vi "Test Flatten.vi"() -> ()   [LabVIEW 2021]
uses:
  ChannelCommon/typedef/FIFO Header.ctl
  ChannelCommon/typedef/Datatype Waveform.ctl
  ChannelCommon/typedef/TimeStamps.ctl
  CIF_NIChn_FIFO_DAQ.lvclass
  D:/dev/Packages/Channel_Manager/src/CIF_NIChn/FIFO_U8/CIF_NIChn_Fifo_U8.lvclass
  D:/dev/Packages/Channel_Manager/src/CIFChannels/CIFChannels.lvclass
  CIFChannels/Typedef/Direction.ctl
  FIFO_U8/CIF_NIChn_Fifo_U8.lvclass/CIF_NIChn_Fifo_U8.ctl
  CIFChannels/CIFChannels.lvclass/CIFChannels.ctl
  <vilib>/CIF Foundation/CIF Utilities/Statistics/I64/Stats_I64_CIF_U.lvclass/Stats_I64_CIF_U.ctl
  CIFChannels/Utilities/Update Flatten Benchmark.vi
  SubVIs/Flatten.vi/587a020d-d764-4ff7-9451-6b801beca2fa.vi
  SubVIs/Flatten.vi/b511efe2-f594-4971-95dc-73ac55586360.vi
  ChannelCommon/CIFFIFO/Flatten/Waveform Flatten.vi
  FIFO_U8/Accessors/Read Payload.vi
  FIFO_U8/Accessors/Write Payload.vi
  SubVIs/Unflatten.vi/4ab41953-a001-49d2-beab-55370b6c3c42.vi
  SubVIs/Unflatten.vi/7cd889b7-face-4678-a9e3-2692853b6930.vi
  ChannelCommon/CIFFIFO/Flatten/Waveform Unflatten.vi
  CIFChannels/Accessors/Write FIFO Timeout.vi
  <vilib>/CIF Foundation/CIF Utilities/Statistics/I64/X1 minus X0.vi
  <vilib>/CIF Foundation/CIF Utilities/Time/System Time/Get System Time.vi
  <vilib>/CIF Foundation/CIF Utilities/DataTypes/Flatten I64.vi
  ChannelCommon/CIFFIFO/Flatten/Waveform Flatten.vi/be24e584-1bb9-4ddb-b1ad-5fa4498d0a1e.vi
  <vilib>/CIF Foundation/CIF Utilities/DataTypes/Flatten U64.vi
  CIFChannels/Utilities/Create Flattened FIFO Header.vi
  ChannelCommon/Utilities/Unflatten Header.vi
  <vilib>/CIF Foundation/CIF Utilities/DataTypes/Unflatten I64.vi
  <vilib>/CIF Foundation/CIF Utilities/Statistics/I64/X1 minus X0.vi/dfabcf33-0dbc-4041-80a5-3dc0c86d2989.vi
  <vilib>/CIF Foundation/CIF Utilities/Time/System Time/LabVIEW Time to TAI Time.vi
  ChannelCommon/CIFFIFO/Flatten/Waveform Flatten.vi/be24e584-1bb9-4ddb-b1ad-5fa4498d0a1e.vi/c28b0ead-42ad-4072-80a2-aca7f2bd7ce3.vi
  ChannelCommon/Utilities/Flatten Header.vi
  CIFChannels/Utilities/Update FIFO Header.vi
  <vilib>/CIF Foundation/CIF Utilities/DataTypes/Unflatten U64.vi
  ChannelCommon/Utilities/Add Error.vi
  <vilib>/CIF Foundation/CIF Utilities/Statistics/I64/X1 minus X0.vi/dfabcf33-0dbc-4041-80a5-3dc0c86d2989.vi/9eb60a9a-770f-4d2d-8b3f-8465c267ecc9.vi
  <vilib>/CIF Foundation/CIF Utilities/Errors/Append Error Location.vi
  CIFChannels/CIFChannels.lvclass
  ChannelCommon/ChannelCommon.lvlib
panel:
  out "Pass":bool
  out "error out":errorcluster
  in  "FIFO Timestamps":T1={"ClockID"=2, "T0"=432, "T_Out"=543}
  out "Data out":T2[](array[typedef])=[{"measurement"=[0.0, 0.0, 0.0, 0.0, 0.0, 0.0, 0.0, 3.14], "dT"=0.01, "Timestamp"=498, "Read Lock"=FALSE}, {"measurement"=[0.0, 0.0, 0.0, 0.0, 0.0, 0.0, 0.0, 9.8], "dT"=0.12, "Timestamp"=12345, "Read Lock"=FALSE}]
  in  "Data In":T2[](array[typedef])=[{"measurement"=[0.0, 0.0, 0.0, 0.0, 0.0, 0.0, 0.0, 3.14], "dT"=0.01, "Timestamp"=498, "Read Lock"=FALSE}, {"measurement"=[0.0, 0.0, 0.0, 0.0, 0.0, 0.0, 0.0, 9.8], "dT"=0.12, "Timestamp"=12345, "Read Lock"=FALSE}]
  out "Header":T3={"Length"=57, "T0"=432, "T_Out"=543, "T_Tx"=1727639110950812000, "Ctr"=1, "ClockID"=2}
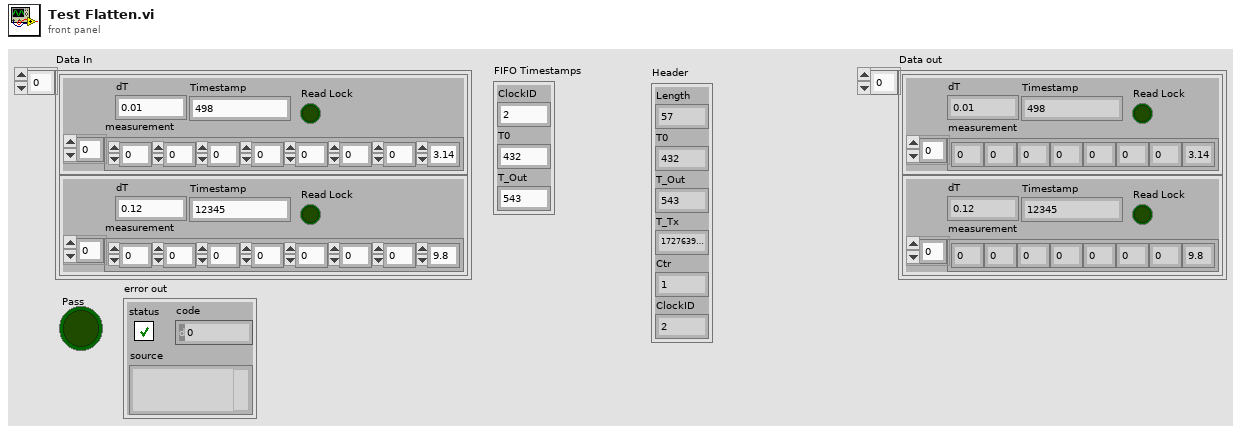
[diagram p1: front panel]
types:
  T1 = typedef "ChannelCommon.lvlib/TimeStamps.ctl" = cluster{"ClockID":u8, "T0":i64, "T_Out":i64}
  T2 = typedef "ChannelCommon.lvlib/Datatype Waveform.ctl" = cluster{"measurement":dbl[], "dT":dbl, "Timestamp":i64, "Read Lock":bool}
  T3 = typedef "ChannelCommon.lvlib/FIFO Header.ctl" = cluster{"Length":u64, "T0":i64, "T_Out":i64, "T_Tx":i64, "Ctr":u64, "ClockID":u8}
  T4 = typedef "CIFChannels.lvclass/Direction.ctl" = enum16{"Publisher", "Subscriber"}
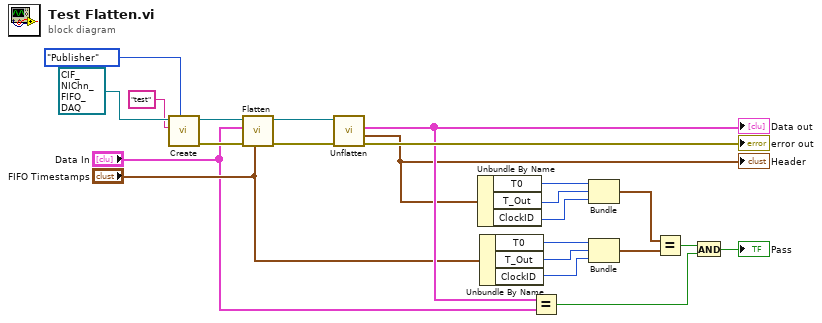
[diagram p0: block diagram]
diagram:
  n1 = call-dynamic "Create.vi"("Direction"=Direction."Publisher", "Name"="test", "CIFFIFO in"=refnum<class "CIF_NIChn_FIFO_DAQ.lvclass"> refnum ("CIF_NIChn_Fifo_Power.lvclass")) -> ("error out"=w17:errorcluster, "CIFFIFO out"=w19:refnum<class "CIF_NIChn_FIFO_DAQ.lvclass">)  [unwired: 7 in]
  n2 = call "Flatten.vi"("FIFO Timestamps"="FIFO Timestamps", "error in (no error)"=w17, "Data In"="Data In", "CIF_NIChn_FIFO_DAQ in"=w19) -> ("error out"=w18:errorcluster, "CIF_NIChn_FIFO_DAQ out"=w23:refnum<class "CIF_NIChn_FIFO_DAQ.lvclass">)  [unwired: 5 in, 1 out]
  n3 = call "Unflatten.vi"("error in (no error)"=w18, "CIF_NIChn_FIFO_DAQ in"=w23) -> ("error out"=→"error out":errorcluster, "Header"=w14:T3, "DAQ Out"=w15:T2[])  [unwired: 6 in, 1 out]
  "Header" <- w14
  "Data out" <- w15
  n4 = Unbundle By Name(w14) -> ("T0"=w12:i64, "T_Out"=w11:i64, "ClockID"=w10:u8)
  n5 = Unbundle By Name("FIFO Timestamps") -> ("T0"=w9:i64, "T_Out"=w8:i64, "ClockID"=w7:u8)
  n6 = Equal?(x=w15, y="Data In") -> (x = y?=w3:bool)
  n7 = Bundle("T0"=w12, "T_Out"=w11, "ClockID"=w10) -> (w5:cluster{"T0":i64, "T_Out":i64, "ClockID":u8})  [unwired: 1 in]
  n8 = Bundle("T0"=w9, "T_Out"=w8, "ClockID"=w7) -> (w6:cluster{"T0":i64, "T_Out":i64, "ClockID":u8})  [unwired: 1 in]
  n9 = Equal?(x=w5, y=w6) -> (x = y?=w4:bool)
  n10 = And(x=w4, y=w3) -> (x .and. y?=→"Pass":bool)
